vi "close.vi"(8 "error in":errorcluster, 11 "module in":refnum<class "RTResourceUtilitzation runtime.lvclass">) -> (0 "error out":errorcluster)   [LabVIEW 2014, in "RTResourceUtilitzation runtime.lvclass"]
doc: "Provides an interface for terminating a module instance. While this interface performs no operations, a child should close and deallocate any open references or memory."
uses:
  RTResourceUtilitzation runtime.lvclass
  RTResourceUtilitzation runtime.lvclass/RTResourceUtilitzation runtime.ctl
  <vilib>/nisyscfg/Close (System).vi
  <vilib>/NI/DCAF/Tag Editor Core/control module/runtime/control module runtime.lvclass
  <vilib>/nisyscfg/nisyscfg.lvlib
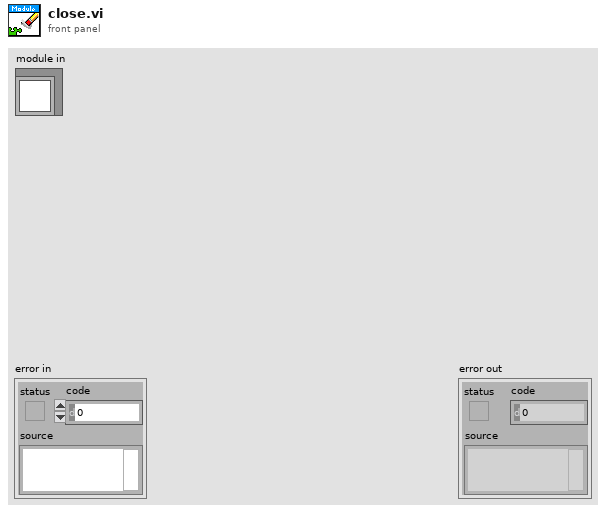
[diagram p1: front panel]
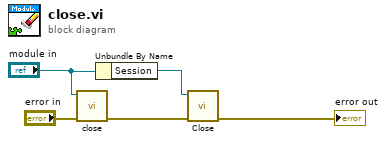
[diagram p0: block diagram]
diagram:
  n1 = call-parent <vilib>:"close.vi"("error in"="error in", "module in"="module in") -> ("error out"=w4:errorcluster)  [unwired: 9 in]
  n2 = Unbundle By Name("module in") -> ("Session"=w1:refnum<k21>)
  n3 = call-poly <vilib>:"Close.vi"("error in (no error)"=w4, "Session in"=w1) -> ("error out"=→"error out":errorcluster)  [unwired: 9 in]
